vi "SE_HV500.constructor.vi"(0 "name":string, 2 "data in":string, 5 "error in(no error)":errorcluster) -> (14 "i ref out":refnum<vi>, 16 "data out":string, 19 "error out":errorcluster)   [LabVIEW 2014, in "SE_HV500.lvlib"]
doc: "High Voltage power supply FUG-HCN. This power supply can deliver upto 65KV. This class uses an instrument driver that is available via http://labview.gsi.de/driver.htm. The device is connected via GPIB. Finally, this device talks to a GPIB driver that must be installed on your system. Whenever a new frequency or amplitude value is set, that value is sent to the DSCInterface process for trending.\n\nauthors: Frank Herfurth (CERN) and Sumit Saxena\nadapted to CS v3 by: R.Savreux, CERN\n\nLicense Agreement for this software:\n\nCopyright (C)\nGesellschaft für Schwerionenforschung, GSI\nPlanckstr. 1\n64291 Darmstadt\nGermany\n\nContact: D.Beck@gsi.de \n\nThis program is free software; you can redistribute it and/or modify it under the terms of the \nGNU General Public License as published by the Free Software Foundation; either version 2 of \nthe license, or (at your option) any later version.\n\nThis program is distributed in the hope that it will be useful, but WITHOUT ANY WARRANTY; \nwithout even the implied warranty of MERCHANTABILITY or FITNESS FOR A PARTICULAR PURPOSE. See the GNU General License for more details (http://www.gnu.org).\n\nGesellschaft für Schwerionenforschung, GSI\nPlanckstr. 1, 64291 Darmstadt, Germany\nFor all questions and ideas contact: M.Richter@gsi.de, H.Brand@gsi.de or D.Beck@gsi.de.\nLast update: 16-JUN-2004"
uses:
  SE_HV500.lvlib
  CSCore/BaseProcess/BaseProcess.lvlib
  CSCore/CSSystem/CSSystemLib/CSSystemLib.lvlib
  CSlibraries-extern/DimLVEvent/LVDimInterface/LVDimInterface.lvlib
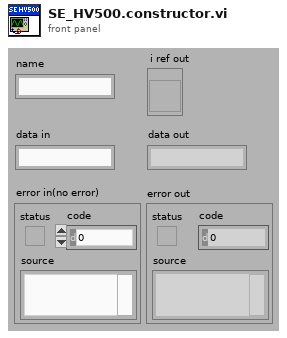
[diagram p1: front panel]
types:
  T1 = enum16{"SetAttribute", "GetAttribute", "CreateAttribute", "DestroyAttribute", "DestroyAllAtributes"}
  T2 = typedef "BaseProcess.lvlib/BaseProcess.i attribute.ctl" = cluster{"EventStatus":string, "EventError":i32, "PresetEvtWatchD":i32, "PresetPdcWatchD":i32, "EventTimeout":i32, "PeriodicInterval":i32, "Interface":string[], "Address":string[], "Special":string[], "PeriodicError":i32, "PeriodicStatus":string, "SuperProc":string, "Descriptors":T3[], "CaseRef":refnum<vi>, "PdcRef":refnum<vi>, "Thread Ref":refnum<vi>, "eventErrorID":i32, "eventStatusID":i32, "periodicErrorID":i32, "periodicStatusID":i32, "pdcCtrID":i32}
  T3 = typedef "BaseProcess.lvlib/BaseProcess.descriptor definition.ctl" = cluster{"selector":string, "descriptor":T4}
  T4 = typedef "BaseProcess.lvlib/BaseProcess.descriptor string definition.ctl" = string
  T5 = typedef "SE_HV500.lvlib/SE_HV500.i attribute.ctl" = cluster{"SetStatus":bool, "Set Voltage":dbl, "VoltageID":i32, "Nom Voltage":dbl, "VISA resource name in":refnum<visa-resource-name>, "Device name":string, "PSRange":i32}
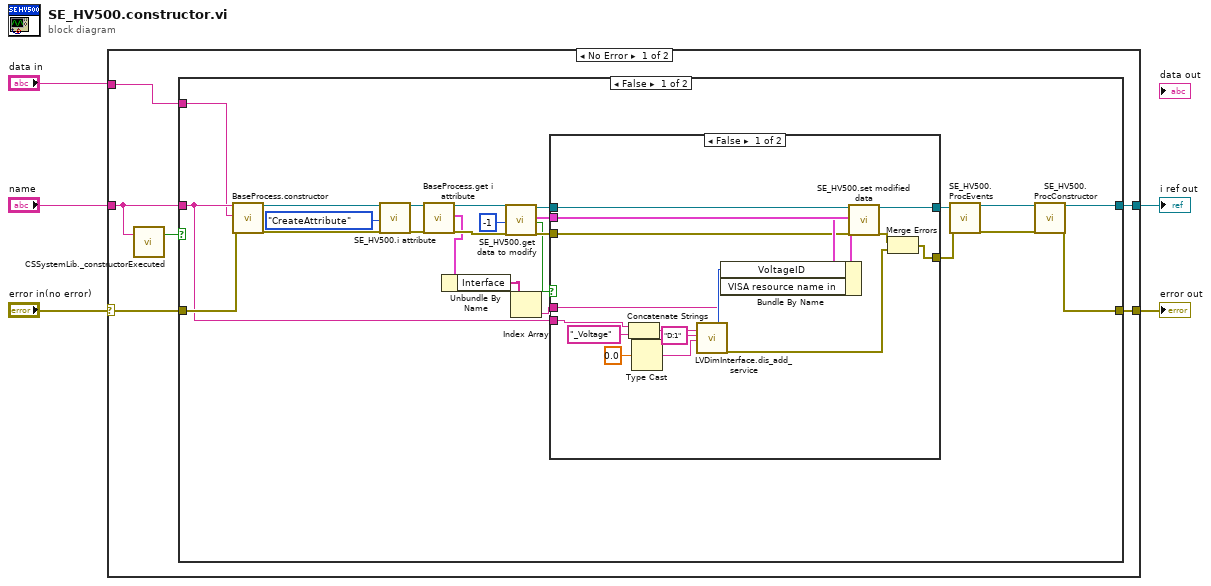
[diagram p0: block diagram]
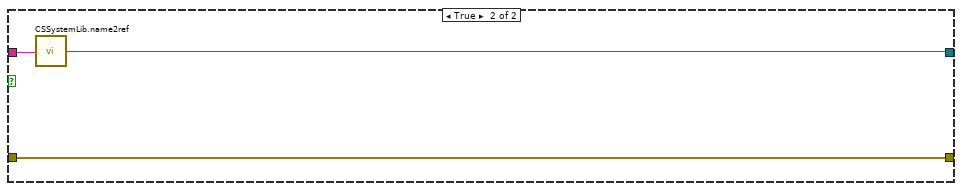
[diagram p3: hidden frame]
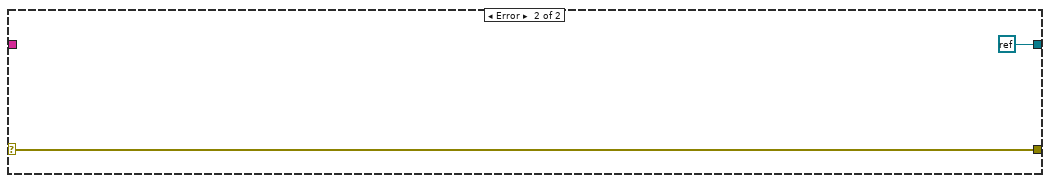
[diagram p4: hidden frame]
diagram:
  n1 = case shown="No Error" "error in(no error)" {
    selector: "error in(no error)" -> [w9 w58]
    tunnel: "name" -> [w8 _]
    tunnel: [w11 refnum<k0> refnum ("i ref out")] -> w4
    tunnel: [w10 w58] -> w3
    tunnel: "data in" -> [w6 _]
    frame No Error {
      n2 = call "CSSystemLib._constructorExecuted.vi"("name"=w8) -> ("constructor executed?"=w7:bool)  [unwired: 18 in]
      n3 = case shown="False" w7 {
        tunnel: [w31 w55] -> w11
        tunnel: [w30 w54] -> w10
        tunnel: w9 -> [w29 w54]
        tunnel: w8 -> [w21 w56]
        tunnel: w6 -> [w20 _]
        frame False {
          n4 = call "BaseProcess.constructor.vi"("name"=w21, "data in"=w20, "error in (no error)"=w29) -> ("i ref out"=w35:refnum<vi>, "error out"=w19:errorcluster)  [unwired: 14 in, 1 out]
          n5 = call "SE_HV500.i attribute.vi"("VI Refnum"=w35, "Action"=T1."CreateAttribute", "error in (no error)"=w19) -> ("VI Refnum out"=w17:refnum<vi>, "error out"=w18:errorcluster)  [unwired: 14 in, 1 out]
          n6 = call "BaseProcess.get i attribute.vi"("i ref in"=w17, "error in (no error)"=w18) -> ("i ref out"=w16:refnum<vi>, "i attribute"=w14:T2, "error out"=w15:errorcluster)  [unwired: 15 in]
          n7 = Unbundle By Name(w14) -> ("Interface"=w13:string[])
          n8 = call "SE_HV500.get data to modify.vi"("i ref in"=w16, "ms timeout (10000)"=-1, "error in (no error)"=w15) -> ("i ref out"=w26:refnum<vi>, "i attribute"=w27:T5, "timed out"=w22:bool, "error out"=w25:errorcluster)  [unwired: 13 in]
          n9 = Index Array(array=w13) -> (element=w12:string)  [unwired: 1 in]
          n10 = case shown="False" w22 {
            tunnel: w27 -> [w51 _]
            tunnel: w26 -> [w50 w53]
            tunnel: w25 -> [w48 w52]
            tunnel: [w47 w53] -> w24
            tunnel: [w45 w52] -> w23
            tunnel: w21 -> [w38 _]
            tunnel: w12 -> [w36 _]
            frame False {
              n11 = Concatenate Strings(w38, "_Voltage" ("string")) -> (w44:string)
              n12 = Type Cast(x=0.0) -> (*(type *) &x=w43:string)  [unwired: 1 in]
              n13 = call "LVDimInterface.dis_add_service.vi"("serviceName"=w44, "typeDescriptor"="D:1", "data"=w43) -> ("my_serviceID"=w39:i32, "error out"=w37:errorcluster)  [unwired: 15 in]
              n14 = Bundle By Name(cluster=w51, "VoltageID"=w39, "VISA resource name in"=w36) -> (w49:T5)
              n15 = call "SE_HV500.set modified data.vi"("i ref in"=w50, "i attribute"=w49, "error in (no error)"=w48) -> ("i ref out"=w47:refnum<vi>, "error out"=w46:errorcluster)  [unwired: 15 in]
              n16 = Merge Errors(w46, w37) -> (w45:errorcluster)
            }
            frame True {
            }
          }
          n17 = call "SE_HV500.ProcEvents.vi"("i ref in"=w24, "error in"=w23) -> ("i ref out"=w33:refnum<vi>, "error out"=w32:errorcluster)  [unwired: 16 in]
          n18 = call "SE_HV500.ProcConstructor.vi"("i ref in"=w33, "error in (no error)"=w32) -> ("i ref out"=w31:refnum<vi>, "error out"=w30:errorcluster)  [unwired: 16 in]
        }
        frame True {
          n19 = call "CSSystemLib.name2ref.vi"("name"=w56) -> ("obj refnum"=w55:refnum<vi>)
        }
      }
    }
    frame Error {
    }
  }
  "i ref out" <- w4
  "error out" <- w3
